vi "eGateHSP_ReadBufferToDoubleArray.vi"(8 "Fehler (Eingang, kein Fehler)":errorcluster, 10 "NumberOfFrames":i32, 11 "e.gate Configuration":T1 {"StartTime" format="%#.10f"; "dActTimeToSecondFactor" format="%#.10f"; "StartTimeToDayFactor" format="%#_10f"}) -> (0 "Fehler (Ausgang)":errorcluster, 3 "Array (Ausgang)":dbl[][](array[numeric]))   [LabVIEW 2016]
uses:
  e.gate Configuration.ctl
  e.gate Channel Data.ctl
  e.gate Data Type.ctl
  e.gate Protocol Type.ctl
  e.gate Module  Data.ctl
  e.gateHSP_DLLhandle.ctl
panel:
  out "channelCount":i32
  out "receivedFrames":i32
  out "complete":i32
  out "Rückgabewert":i32
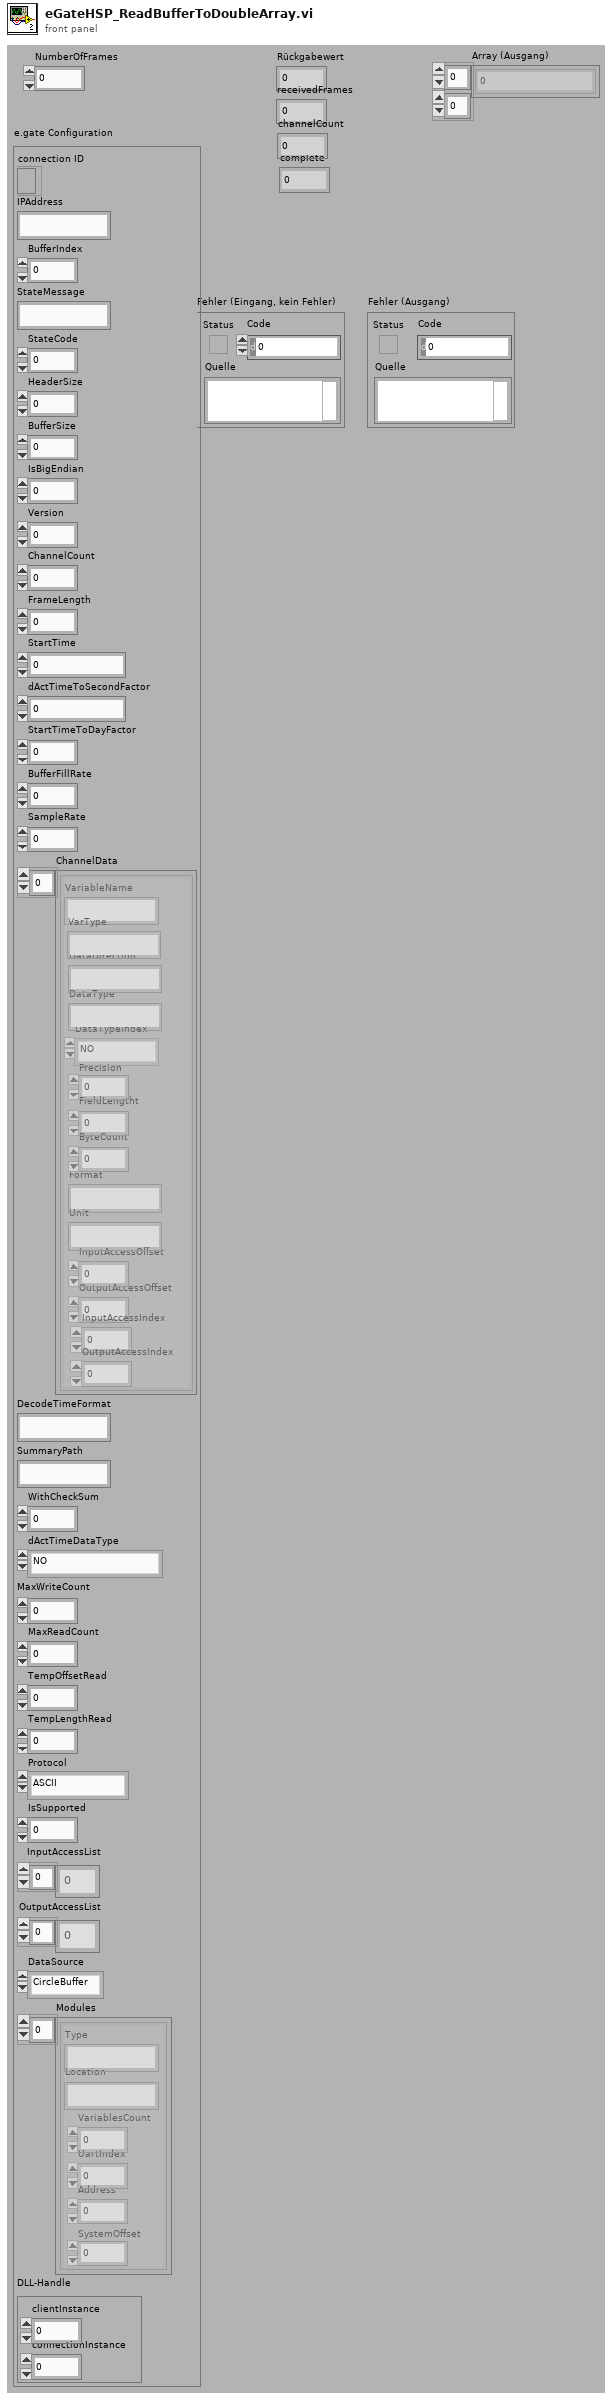
[diagram p1: front panel]
types:
  T1 = typedef "e.gate Configuration.ctl" = cluster{"connection ID":refnum<k5>, "IPAddress":string, "BufferIndex":i32, "StateMessage":string, "StateCode":i8, "HeaderSize":i32, "BufferSize":i32, "IsBigEndian":i32, "Version":i32, "ChannelCount":i32, "FrameLength":i32, "StartTime":dbl, "dActTimeToSecondFactor":dbl, "StartTimeToDayFactor":dbl, "BufferFillRate":dbl, "SampleRate":dbl, "ChannelData":T2[], "DecodeTimeFormat":string, "SummaryPath":string, "WithCheckSum":i32, "dActTimeDataType":T3, "MaxWriteCount":i32, "MaxReadCount":i32, "TempOffsetRead":i32, "TempLengthRead":i32, "Protocol":T4, "IsSupported":i32, "InputAccessList":i32[], "OutputAccessList":i32[], "DataSource":enum16{"CircleBuffer", "test.con Logger", "test.con Archive"}, "Modules":T5[], "DLL-Handle":T6}
  T2 = typedef "e.gate Channel Data.ctl" = cluster{"VariableName":string, "DataDirection":string, "DataType":string, "DataTypeIndex":T3, "Precision":i16, "FieldLengtht":i16, "ByteCount":i32, "Format":string, "Unit":string, "InputAccessOffset":i32, "OutputAccessOffset":i16, "InputAccessIndex":i16, "OutputAccessIndex":i16, "VarType":string}
  T3 = typedef "e.gate Data Type.ctl" = enum16{"NO", "BOOL", "SINT8", "USINT8", "SINT16", "USINT16", "SINT32", "USINT32", "FLOAT", "SET8", "SET16", "SET32", "DOUBLE", "SINT64", "USINT64", "SET64"}
  T4 = typedef "e.gate Protocol Type.ctl" = enum16{"ASCII", "HighspeedPort Online", "HighspeedPort Buffer", "eGateHighspeedPortDLL "}
  T5 = typedef "e.gate Module  Data.ctl" = cluster{"Type":string, "Location":string, "VariablesCount":i16, "UartIndex":i16, "Address":i16, "SystemOffset":i16}
  T6 = typedef "e.gateHSP_DLLhandle.ctl" = cluster{"clientInstance":i32, "connectionInstance":i32}
  T7 = cluster{"HighSpeedPort":path, "Utility":path, "Ismbus32":path}
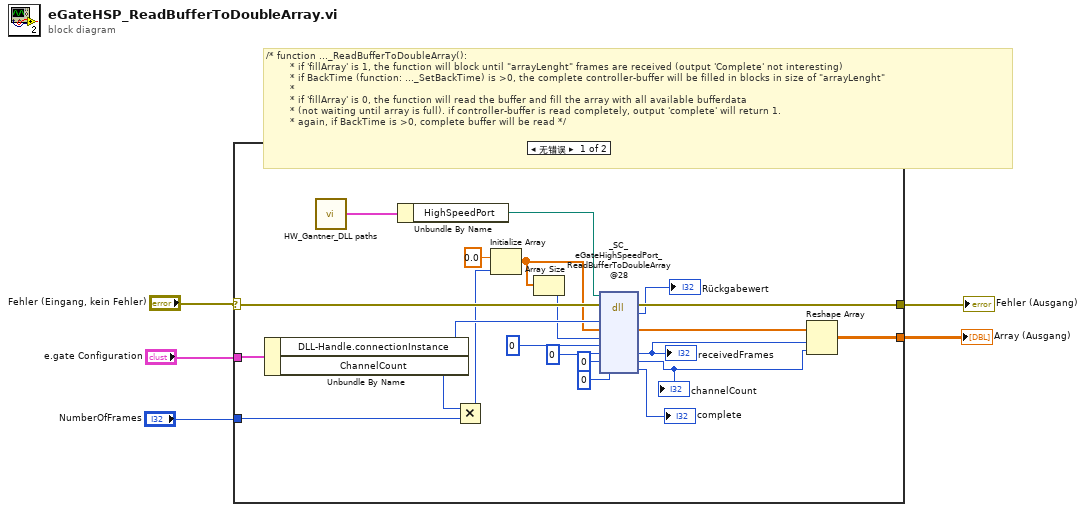
[diagram p0: block diagram]
diagram:
  # "/* function ..._ReadBufferToDoubleArray():\n        * if 'fillArray' is 1, the function will block until \"arrayLenght\" frames are received (output 'Complete' not interesting)\n        * if BackTime (function: ..._SetBackTime) is >0, the complete controller-buffer will be filled in blocks in size of \"arrayLenght\"\n        * \n        * if 'fillArray' is 0, the function will read the buffer and fill the array with all available bufferdata\n        * (not waiting until array is full). if controller-buffer is read completely, output 'complete' will return 1.\n        * again, if BackTime is >0, complete buffer will be read */"
  n1 = case shown="无错误" "Fehler (Eingang, kein Fehler)" {
    selector: "Fehler (Eingang, kein Fehler)" -> [w24 w28]
    tunnel: "e.gate Configuration" -> [w27 _]
    tunnel: [w26 w28] -> w3
    tunnel: "NumberOfFrames" -> [w19 _]
    tunnel: [w10 _] -> w1
    frame No Error {
      n2 = Unbundle By Name(w27) -> ("DLL-Handle.connectionInstance"=w23:i32, "ChannelCount"=w20:i32)
      n3 = call "HW_Gantner_DLL paths.vi"() -> ("DLL paths"=w7:T7)  [unwired: 11 in]
      n4 = Unbundle By Name(w7) -> ("HighSpeedPort"=w6:path)
      n5 = Multiply(x=w20, y=w19) -> (x*y=w17:i32)
      n6 = Initialize Array(0.0 ("Element"), w17) -> (w16:dbl[])
      n7 = Array Size(array=w16) -> (size(s)=w15:i32)
      n8 = dll-call lib="E:/Projects/16S005 C5SF  - QinLei/5#/SourceCodes 160905/ZC141227/Gantner/GantnerDLL/eGateHighSpeedPort.dll" fn="_SC_eGateHighSpeedPort_ReadBufferToDoubleArray@28"(path in=w6, error in=w24, "connectionInstance"=w23, "valueArray"=w16, "arrayLength"=w15, "fillArray"=0, "receivedFrames"=0, "channelCount"=0, "complete"=0) -> (error out=w26:errorcluster, "Rückgabewert"=→"Rückgabewert":i32, "valueArray"=w11:dbl[], "receivedFrames"=w9:i32, "channelCount"=w8:i32, "complete"=→"complete":i32)  [unwired: 4 in, 1 out]
      "receivedFrames" <- w9
      "channelCount" <- w8
      n9 = Reshape Array(w11, w9, w8) -> (w10:dbl[][])
    }
    frame Error {
    }
  }
  "Fehler (Ausgang)" <- w3
  "Array (Ausgang)" <- w1
